vi "Create from Known Hosts.vi"(8 "Error In":errorcluster, 11 "Known Hosts In":refnum<class "KnownHosts.lvclass">) -> (0 "Error Out":errorcluster, 2 "Known Host":refnum<class "KnownHost.lvclass">, 3 "Known Hosts Out":refnum<class "KnownHosts.lvclass">)   [LabVIEW 2018, in "Toolkit.lvlib" / "KnownHost.lvclass"]
uses:
  KnownHost.lvclass
  KnownHosts/KnownHosts.lvclass
  KnownHosts/KnownHosts.lvclass/KnownHosts.ctl
  Session/Session.lvclass/Session.ctl
  SSH/SSH.lvclass
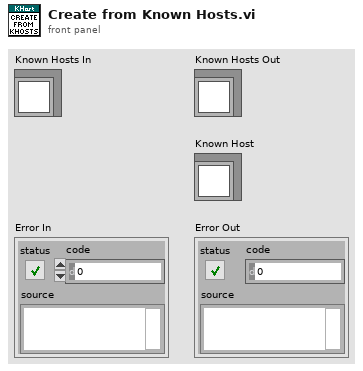
[diagram p1: front panel]
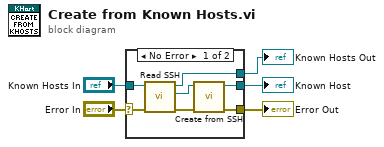
[diagram p0: block diagram]
diagram:
  n1 = case shown="No Error" "Error In" {
    selector: "Error In" -> [w11 w14]
    tunnel: [w8 w14] -> w4
    tunnel: [w7 _] -> w3
    tunnel: "Known Hosts In" -> [w12 w13]
    tunnel: [w6 w13] -> w1
    frame No Error {
      n2 = call "Read SSH.vi"("Error In"=w11, "Known Hosts In"=w12) -> ("Error Out"=w9:errorcluster, "SSH"=w10:refnum<class "SSH.lvclass">, "Known Hosts Out"=w6:refnum<class "KnownHosts.lvclass">)  [unwired: 7 in]
      n3 = call "Create from SSH.vi"("Error In"=w9, "SSH"=w10) -> ("Error Out"=w8:errorcluster, "Known Host"=w7:refnum<class "KnownHost.lvclass">)  [unwired: 8 in]
    }
    frame Error {
    }
  }
  "Error Out" <- w4
  "Known Host" <- w3
  "Known Hosts Out" <- w1
